vi "LSCI332CurveHandler.vi"(0 "VISA Rsrc":refnum<visa-resource-name>="GPIB1::12::INSTR" caption="Adresse du contrôlleur", 2 "No Courbe":u32=21 min=1 max=41 step=1, 3 "Nom":string="CourbeTest", 4 "No de série":string="Standard", 5 "Start path":path=path "C:/Donnees/Courbes de calibration de Temp" caption="Répertoire Initiale", 6 "Coefficient":u16(ring) items=["Faites un choix", "négatif", "positif"], 10 "Table":string[][](table) caption="Table de Calibration", 11 "error in":errorcluster, 13 "TLim":dbl=475.0 caption="T° de Contrôle Max (K)", 14 "Format":u16(ring) items=["Faites un choix", "mV/K", "V/K", "Ohm/K", "log Ohm/K"]) -> (15 "error out":errorcluster)   [LabVIEW 2019]
doc: "Ce Vipermet la gestion des données de calibration du contrôlleur. Les données peuvent être lu ou écrit de celui-ci et sauvegardées dans un fichier texte, qui peut être ouvert par la suite."
uses:
  <vilib>/Utility/error.llb/DialogType.ctl
panel:
  out "Courbe Calib":string[][](table) caption="Courbes de Calibration"
  in  "EffCont":bool
  out "BUSY":bool caption="Opération en cours"
  in  "SauvCont":bool
  in  "ÉcrireCont":bool
  in  "LireCont":bool
  in  "ÉcrireFich":bool
  in  "LireFich":bool
  in  "Quit":bool
  # "Courbe d'un\nFichier"
  # "+5"
  # "Courbe du\nContrôlleur"
  # "+10"
  # "+15"
  # "+20"
  # "Max 200 lignes. \"Capteur\" doit être en ordre croissant"
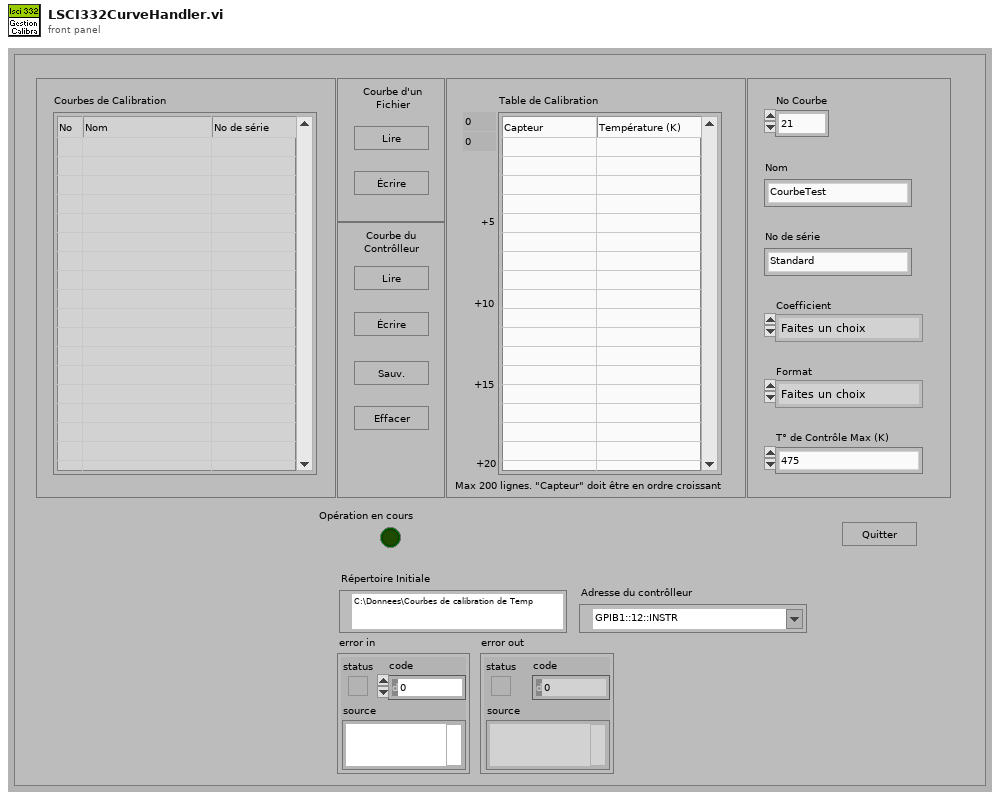
[diagram p1: front panel]
types:
  T1 = typedef "DialogType.ctl" = u16
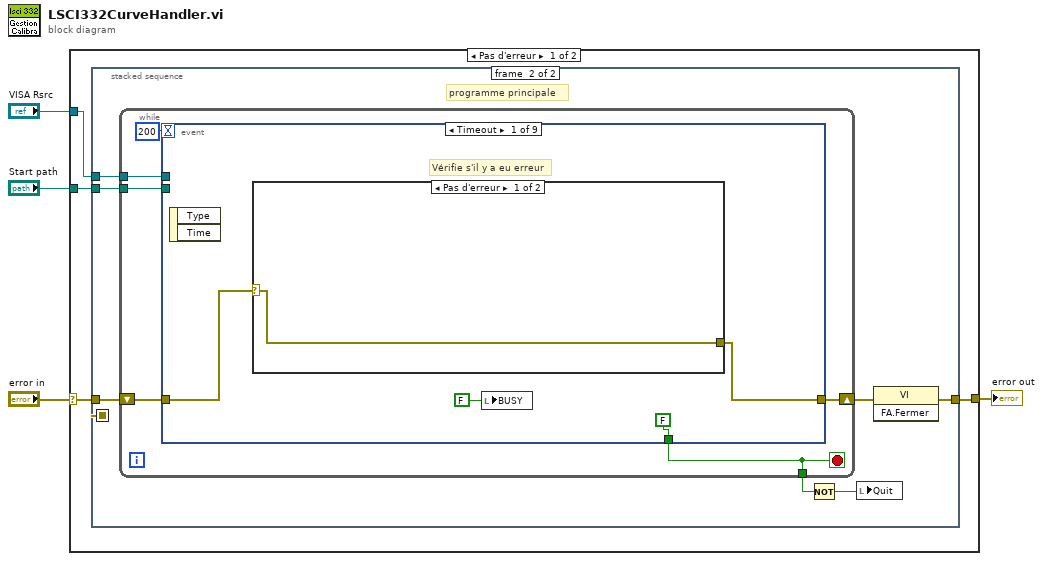
[diagram p0: block diagram]
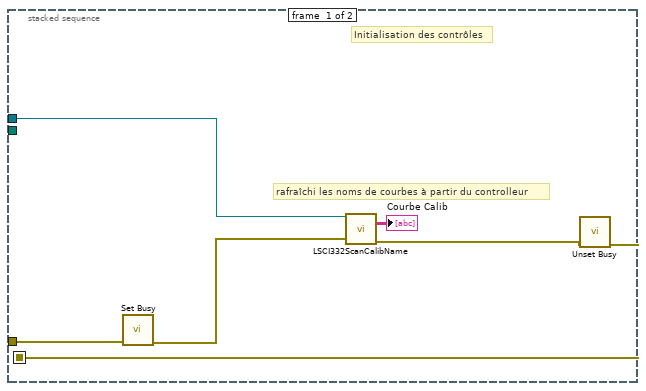
[diagram p2: hidden frame]
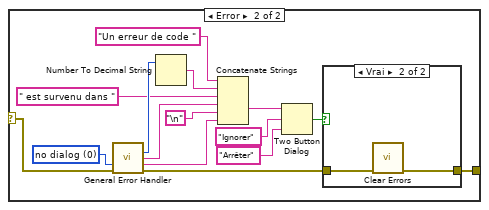
[diagram p3: hidden frame]
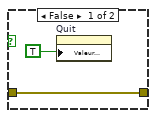
[diagram p4: hidden frame]
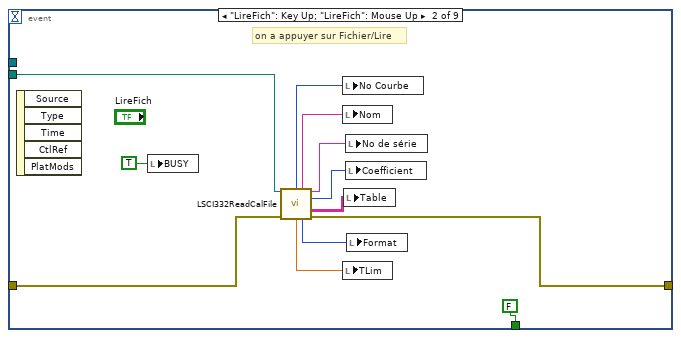
[diagram p5: hidden frame]
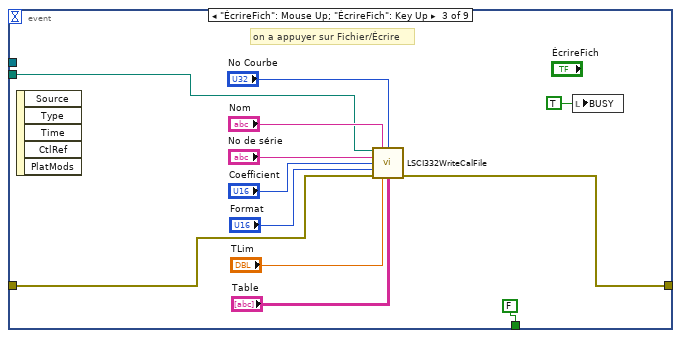
[diagram p6: hidden frame]
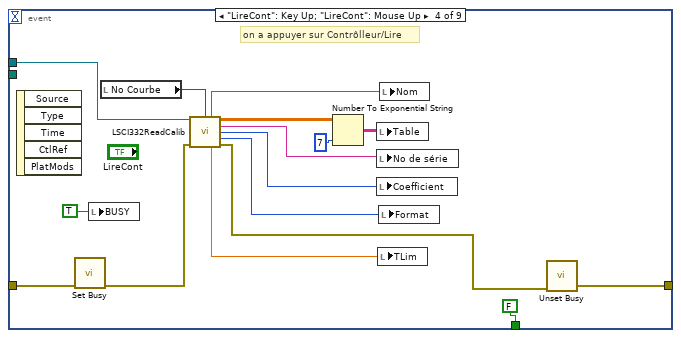
[diagram p7: hidden frame]
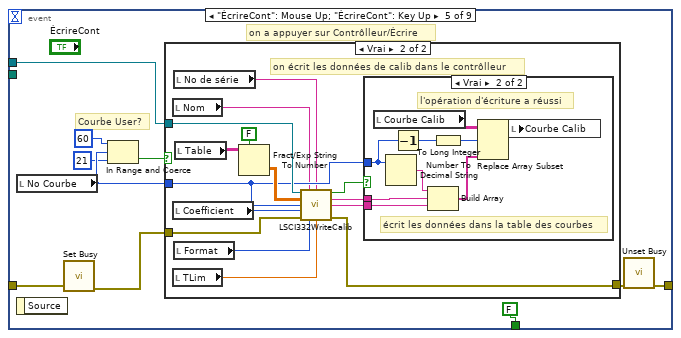
[diagram p8: hidden frame]
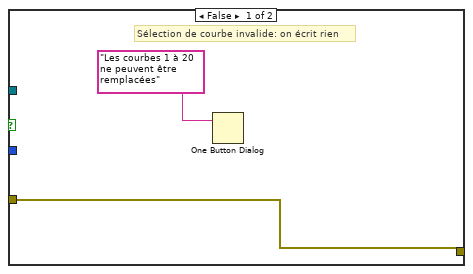
[diagram p9: hidden frame]
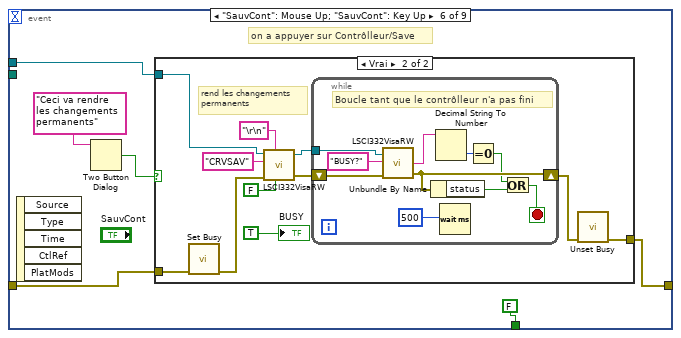
[diagram p11: hidden frame]
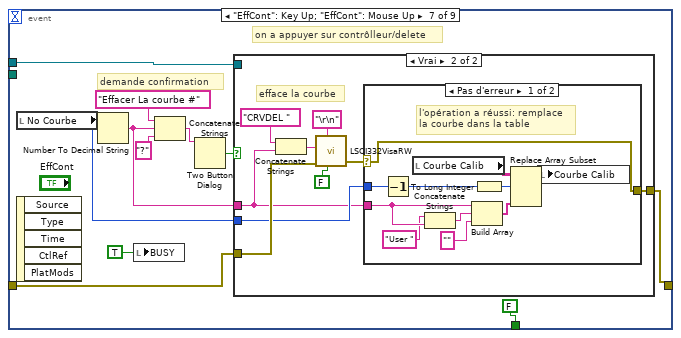
[diagram p13: hidden frame]
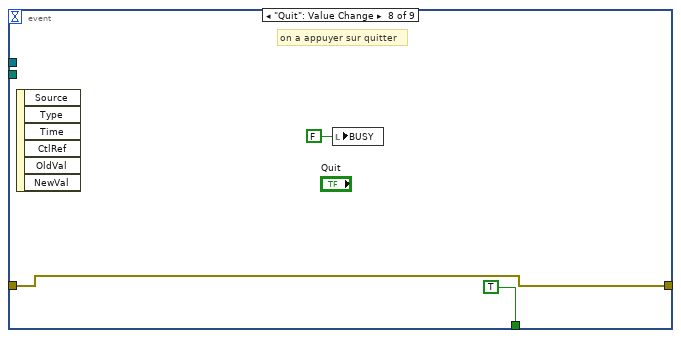
[diagram p16: hidden frame]
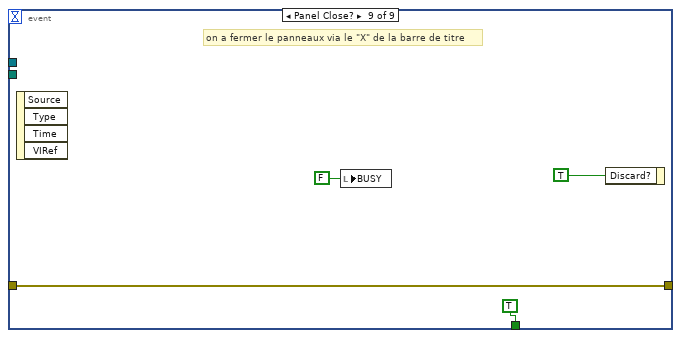
[diagram p17: hidden frame]
diagram:
  n1 = case shown="Pas d'erreur" "error in" {
    selector: "error in" -> [w7 w196]
    tunnel: [w5 w196] -> w3
    tunnel: "Start path" -> [w8 _]
    tunnel: "VISA Rsrc" -> [w6 _]
    frame No Error {
      n2 = stacked-sequence {
        seq-local: [w9 _] -> [_ w17]
        tunnel: w8 -> [_ w21]
        tunnel: w7 -> [w12 _]
        tunnel: w6 -> [w13 w20]
        tunnel: [_ w15] -> w5
        frame #0 {
          # "rafraîchi les noms de courbes à partir du controlleur"
          # "Initialisation des contrôles"
          n3 = call <vilib>:"Set Busy.vi"("error in (no error)"=w12) -> ("error out"=w11:errorcluster)  [unwired: 9 in, 1 out]
          n4 = call <userlib>:"LSCI332ScanCalibName.vi"("VISA Rsrc"=w13, "error in"=w11) -> ("Courbe Calib"=→"Courbe Calib":string[][], "error out"=w10:errorcluster)  [unwired: 12 in]
          n5 = call <vilib>:"Unset Busy.vi"("error in (no error)"=w10) -> ("error out"=w9:errorcluster)  [unwired: 10 in]
        }
        frame #1 {
          # "programme principale"
          n6 = while {
            tunnel: w21 -> [w26]
            shift-right: [w24] -> w16
            shift-left: w17 -> [w25]
            tunnel: w20 -> [w23]
            tunnel: [w22] -> w19
            stop <- w22 stop-if-true
            n7 = event shown="[0] Timeout" {
              selector: _ -> [_ _ _ _ _ _ _ _ _]
              dyn-events: _ -> [_ _ _ _ _ _ _ _ _]
              timeout: 200 -> [_ _ _ _ _ _ _ _ _]
              tunnel: w26 -> [_ w63 w64 _ _ _ _ _ _]
              tunnel: w25 -> [w30 w62 w65 w81 w98 w133 w160 w190 w193]
              tunnel: [w29 w61 w69 w79 w99 w132 w157 w190 w193] -> w24
              tunnel: w23 -> [_ _ _ w91 w101 w130 w166 _ _]
              tunnel: [FALSE FALSE FALSE FALSE FALSE FALSE FALSE TRUE TRUE] -> w22
              event Timeout {
                # "Vérifie s'il y a eu erreur"
                n8 = event-data() -> ()  [unwired: 1 in, 2 out]
                n9 = case shown="Pas d'erreur" w30 {
                  selector: w30 -> [w32 w33]
                  tunnel: [w32 w34] -> w29
                  frame No Error {
                  }
                  frame Error {
                    w44 = T1 0 items=["no dialog", "OK message", "continue or stop message", "OK message + warnings", "continue/stop + warnings"] ("type of dialog (OK msg:1)")
                    n10 = call <vilib>:"General Error Handler.vi"("type of dialog (OK msg:1)"=w44, "error in (no error)"=w33) -> ("code out"=w40:i32, "source out"=w39:string, "message"=w37:string, "error out"=w35:errorcluster)  [unwired: 9 in, 1 out]
                    n11 = Number To Decimal String(number=w40) -> (decimal integer string=w41:string)  [unwired: 1 in]
                    n12 = Concatenate Strings("Un erreur de code " ("string"), w41, " est survenu dans " ("string"), w39, "\n", w37) -> (w36:string)
                    n13 = Two Button Dialog(message=w36, 1:"Arrêter" ("F button name (\"Cancel\")"), 2:"Ignorer" ("T button name (\"OK\")")) -> (T button?=w47:bool)
                    n14 = case shown="Vrai" w47 {
                      tunnel: w35 -> [w49 w50]
                      tunnel: [w49 w51] -> w34
                      frame False {
                        n15 = property on="Quit" class="Bool (strict)"("Valeur (Signalisation)"=TRUE ("Value (Signaling)")) -> ()  [unwired: 2 in, 2 out]
                      }
                      frame True {
                        n16 = call <vilib>:"Clear Errors.vi"("error in (no error)"=w50) -> ("error out"=w51:errorcluster)  [unwired: 5 in, 1 out]
                      }
                    }
                  }
                }
                n17 = local write "BUSY"(FALSE ("BUSY")) -> ()
              }
              event "LireFich": Key Up; "LireFich": Mouse Up {
                # "on a appuyer sur Fichier/Lire"
                n18 = event-data() -> ()  [unwired: 1 in, 5 out]
                n19 = local write "BUSY"(TRUE ("BUSY")) -> ()
                n20 = call <userlib>:"LSCI332ReadCalFile.vi"("Start path"=w63, "error in"=w62) -> ("No Courbe"=w55:u32, "Nom"=w54:string, "No de série"=w58:string, "Coefficient"=w59:u16, "Table"=w60:string[][], "TLim"=w57:dbl, "Format"=w56:u16, "error out"=w61:errorcluster)  [unwired: 6 in]
                n21 = local write "No Courbe"(w55) -> ()
                n22 = local write "Nom"(w54) -> ()
                n23 = local write "TLim"(w57) -> ()
                n24 = local write "Table"(w60) -> ()
                n25 = local write "No de série"(w58) -> ()
                n26 = local write "Coefficient"(w59) -> ()
                n27 = local write "Format"(w56) -> ()
              }
              event "ÉcrireFich": Mouse Up; "ÉcrireFich": Key Up {
                # "on a appuyer sur Fichier/Écrire"
                n28 = event-data() -> ()  [unwired: 1 in, 5 out]
                n29 = call <userlib>:"LSCI332WriteCalFile.vi"("Start path"=w64, "Nom"="Nom", "No Courbe"="No Courbe", "No de série"="No de série", "Coefficient"="Coefficient", "Format"="Format", "error in"=w65, "TLim"="TLim", "Table"="Table") -> ("error out"=w69:errorcluster)  [unwired: 6 in]
                n30 = local write "BUSY"(TRUE ("BUSY")) -> ()
              }
              event "LireCont": Key Up; "LireCont": Mouse Up {
                # "on a appuyer sur Contrôlleur/Lire"
                n31 = event-data() -> ()  [unwired: 1 in, 5 out]
                n32 = call <vilib>:"Set Busy.vi"("error in (no error)"=w81) -> ("error out"=w80:errorcluster)  [unwired: 9 in, 1 out]
                n33 = local write "BUSY"(TRUE ("BUSY")) -> ()
                n34 = local read "No Courbe"() -> (w89:u32)
                n35 = call <userlib>:"LSCI332ReadCalib.vi"("VISA Rsrc"=w91, "No Courbe"=w89, "error in"=w80) -> ("Nom"=w90:string, "ValCalib"=w87:dbl[][], "No de série"=w85:string, "Coefficient"=w84:u16, "Format"=w83:u16, "TLim"=w82:dbl, "error out"=w78:errorcluster)  [unwired: 6 in]
                n36 = Number To Exponential String(number=w87, precision (6)=7) -> (E-format string=w86:string[][])  [unwired: 2 in]
                n37 = local write "Table"(w86) -> ()
                n38 = local write "No de série"(w85) -> ()
                n39 = local write "Coefficient"(w84) -> ()
                n40 = local write "TLim"(w82) -> ()
                n41 = local write "Format"(w83) -> ()
                n42 = local write "Nom"(w90) -> ()
                n43 = call <vilib>:"Unset Busy.vi"("error in (no error)"=w78) -> ("error out"=w79:errorcluster)  [unwired: 10 in]
              }
              event "ÉcrireCont": Mouse Up; "ÉcrireCont": Key Up {
                # "Courbe User?"
                # "on a appuyer sur Contrôlleur/Écrire"
                n44 = local read "No Courbe"() -> (w95:u32)
                n45 = event-data() -> ()  [unwired: 1 in, 1 out]
                n46 = call <vilib>:"Set Busy.vi"("error in (no error)"=w98) -> ("error out"=w97:errorcluster)  [unwired: 9 in, 1 out]
                n47 = In Range and Coerce(upper limit=u32 60, x=w95, lower limit=u32 21) -> (In Range?=w92:bool)  [unwired: 1 out]
                n48 = case shown="Vrai" w92 {
                  tunnel: w95 -> [_ w109]
                  tunnel: w101 -> [_ w114]
                  tunnel: [w102 w111] -> w100
                  tunnel: w97 -> [w102 w110]
                  frame False {
                    # "Sélection de courbe invalide: on écrit rien"
                    n49 = One Button Dialog(message="Les courbes 1 à 20 ne peuvent être remplacées") -> ()  [unwired: 1 in, 1 out]
                  }
                  frame True {
                    # "on écrit les données de calib dans le contrôlleur"
                    n50 = local read "Nom"() -> (w108:string)
                    n51 = local read "Coefficient"() -> (w118:u16)
                    n52 = local read "TLim"() -> (w112:dbl)
                    n53 = local read "No de série"() -> (w107:string)
                    n54 = local read "Format"() -> (w113:u16)
                    n55 = local read "Table"() -> (w117:string[][])
                    n56 = Fract/Exp String To Number(use system decimal point (T)=FALSE, string=w117) -> (number=w116:dbl[][])  [unwired: 2 in, 1 out]
                    n57 = call <userlib>:"LSCI332WriteCalib.vi"("VISA Rsrc"=w114, "Nom"=w108, "No de série"=w107, "ValCalib"=w116, "No Courbe"=w109, "Coefficient"=w118, "error in"=w110, "Format"=w113, "TLim"=w112) -> ("Complété"=w104:bool, "Nom Out"=w106:string, "No de série Out"=w105:string, "error out"=w111:errorcluster)  [unwired: 3 in]
                    n58 = case shown="Vrai" w104 {
                      tunnel: w109 -> [_ w121]
                      tunnel: w106 -> [_ w125]
                      tunnel: w105 -> [_ w124]
                      frame False {
                        # "l'opération d'écriture a échoué"
                      }
                      frame True {
                        # "l'opération d'écriture a réussi"
                        # "écrit les données dans la table des courbes"
                        n59 = local read "Courbe Calib"() -> (w120:string[][])
                        n60 = Number To Decimal String(number=w121) -> (decimal integer string=w126:string)  [unwired: 1 in]
                        n61 = Decrement(x=w121) -> (x-1=w119:u32)
                        n62 = Build Array(w126, w125, w124) -> (w123:string[])
                        n63 = To Long Integer(number=w119) -> (32bit integer=w127:i32)
                        n64 = Replace Array Subset(array=w120, new element=w123, index (row)=w127) -> (w122:string[][])  [unwired: 1 in]
                        n65 = local write "Courbe Calib"(w122) -> ()
                      }
                    }
                  }
                }
                n66 = call <vilib>:"Unset Busy.vi"("error in (no error)"=w100) -> ("error out"=w99:errorcluster)  [unwired: 10 in]
              }
              event "SauvCont": Mouse Up; "SauvCont": Key Up {
                # "on a appuyer sur Contrôlleur/Save"
                n67 = event-data() -> ()  [unwired: 1 in, 5 out]
                n68 = Two Button Dialog(message="Ceci va rendre les changements permanents") -> (T button?=w129:bool)  [unwired: 2 in]
                n69 = case shown="Vrai" w129 {
                  tunnel: w133 -> [w134 w139]
                  tunnel: [w134 w137] -> w132
                  tunnel: w130 -> [_ w135]
                  frame False {
                    # "opération annulée"
                  }
                  frame True {
                    # "rend les changements permanents"
                    n70 = call <vilib>:"Set Busy.vi"("error in (no error)"=w139) -> ("error out"=w138:errorcluster)  [unwired: 9 in, 1 out]
                    n71 = call <userlib>:"LSCI332VisaRW.vi"("Lecture?(T)"=FALSE, "error in (no error)"=w138, "EOS (Aucun)"="\r\n", "ChaineCom"="CRVSAV", "VISA Rsrc"=w135) -> ("error out"=w141:errorcluster, "VISA Rsrc Out"=w142:refnum<visa-resource-name>)  [unwired: 2 in, 2 out]
                    n72 = while {
                      shift-right: [w149] -> w136
                      shift-left: w141 -> [w153]
                      tunnel: w142 -> [w150]
                      stop <- w148 stop-if-true
                      # "Boucle tant que le contrôlleur n'a pas fini"
                      n73 = call <userlib>:"LSCI332VisaRW.vi"("error in (no error)"=w153, "ChaineCom"="BUSY?", "VISA Rsrc"=w150) -> ("error out"=w149:errorcluster, "ChaineRep"=w151:string)  [unwired: 4 in, 2 out]
                      n74 = Unbundle By Name(w149) -> ("status"=w147:bool)
                      n75 = Decimal String To Number(string=w151) -> (number=w152:i32)  [unwired: 2 in, 1 out]
                      n76 = Wait (ms)(milliseconds to wait=u32 500) -> ()  [unwired: 1 out]
                      n77 = Equal To 0?(x=w152) -> (x = 0?=w146:bool)
                      n78 = Or(x=w146, y=w147) -> (x .or. y?=w148:bool)
                    }
                    n79 = call <vilib>:"Unset Busy.vi"("error in (no error)"=w136) -> ("error out"=w137:errorcluster)  [unwired: 10 in]
                    "BUSY" <- TRUE ("BUSY")
                  }
                }
              }
              event "EffCont": Key Up; "EffCont": Mouse Up {
                # "demande confirmation"
                # "on a appuyer sur contrôlleur/delete"
                n80 = local read "No Courbe"() -> (w158:u32)
                n81 = event-data() -> ()  [unwired: 1 in, 5 out]
                n82 = Number To Decimal String(number=w158) -> (decimal integer string=w161:string)  [unwired: 1 in]
                n83 = local write "BUSY"(TRUE ("BUSY")) -> ()
                n84 = Concatenate Strings("Effacer La courbe #" ("message"), w161, "?") -> (w162:string)
                n85 = Two Button Dialog(message=w162) -> (T button?=w165:bool)  [unwired: 2 in]
                n86 = case shown="Vrai" w165 {
                  tunnel: w166 -> [_ _]
                  tunnel: w161 -> [_ w170]
                  tunnel: w160 -> [w167 w172]
                  tunnel: w158 -> [_ w171]
                  tunnel: [w167 w168] -> w157
                  frame False {
                  }
                  frame True {
                    # "efface la courbe"
                    n87 = Concatenate Strings("CRVDEL ", w170) -> (w176:string)
                    n88 = call <userlib>:"LSCI332VisaRW.vi"("Lecture?(T)"=FALSE, "error in (no error)"=w172, "EOS (Aucun)"="\r\n", "ChaineCom"=w176) -> ("error out"=w169:errorcluster)  [unwired: 3 in, 3 out]
                    n89 = case shown="Pas d'erreur" w169 {
                      selector: w169 -> [w177 w188]
                      tunnel: w171 -> [w187 _]
                      tunnel: w170 -> [w182 _]
                      tunnel: [w177 w188] -> w168
                      frame No Error {
                        # "l'opération a réussi: remplace la courbe dans la table"
                        n90 = Decrement(x=w187) -> (x-1=w183:u32)
                        n91 = local read "Courbe Calib"() -> (w184:string[][])
                        n92 = Concatenate Strings("User " ("string"), w182) -> (w179:string)
                        n93 = Build Array(w182, w179, "" ("element")) -> (w181:string[])
                        n94 = To Long Integer(number=w183) -> (32bit integer=w186:i32)
                        n95 = Replace Array Subset(array=w184, new element=w181, index (row)=w186) -> (w185:string[][])  [unwired: 1 in]
                        n96 = local write "Courbe Calib"(w185) -> ()
                      }
                      frame Error {
                        # "l'opération a échoué"
                      }
                    }
                  }
                }
              }
              event "Quit": Value Change {
                # "on a appuyer sur quitter"
                n97 = event-data() -> ()  [unwired: 1 in, 6 out]
                n98 = local write "BUSY"(FALSE ("BUSY")) -> ()
              }
              event Panel Close? {
                # "on a fermer le panneaux via le \"X\" de la barre de titre"
                n99 = event-data() -> ()  [unwired: 1 in, 4 out]
                n100 = local write "BUSY"(FALSE ("BUSY")) -> ()
                n101 = event-data("Discard?"=TRUE) -> ()  [unwired: 1 in, 1 out]
              }
            }
          }
          n102 = Not(x=w19) -> (.not. x?=w18:bool)
          n103 = local write "Quit"(w18) -> ()
          n104 = invoke class="VI" method="FA.Fermer"(error in=w16) -> (error out=w15:errorcluster)  [unwired: 2 in, 2 out]
        }
      }
    }
    frame Error {
    }
  }
  "error out" <- w3
